vi "List ST-Link Infors.vi"(8 "error in (no error)":errorcluster) -> (0 "error out":errorcluster, 2 "Number":i32, 3 "ST-Links":cluster{"SN":string, "FW":string}[](array[cluster]))   [LabVIEW 2015, in "ST-Link.lvlib"]
doc: "识别已连接的ST-Link烧录器，返回连接数量，并获取其SN和FW版本信息。\n\n[ST-Links]: 簇数组，簇中包含两个元素。\n -->SN: 烧录器的SN；\n --> FW: 烧录器的固件版本；\n[Number]: 返回连接的烧录器数量。"
uses:
  ST-Link.lvlib
panel:
  out "standard output":string
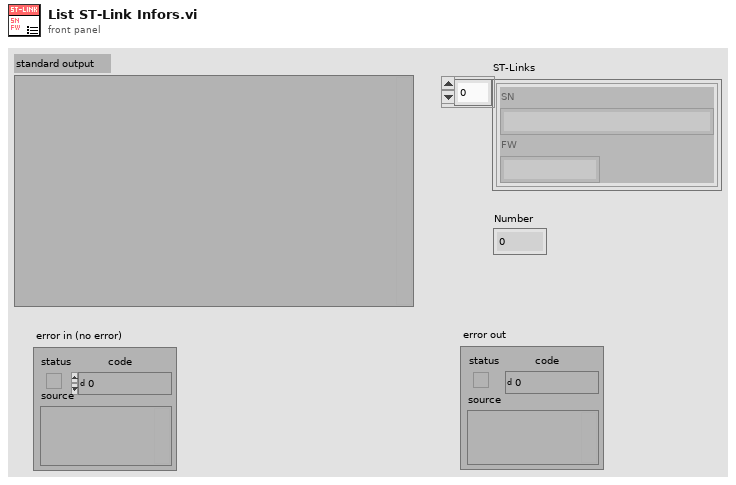
[diagram p1: front panel]
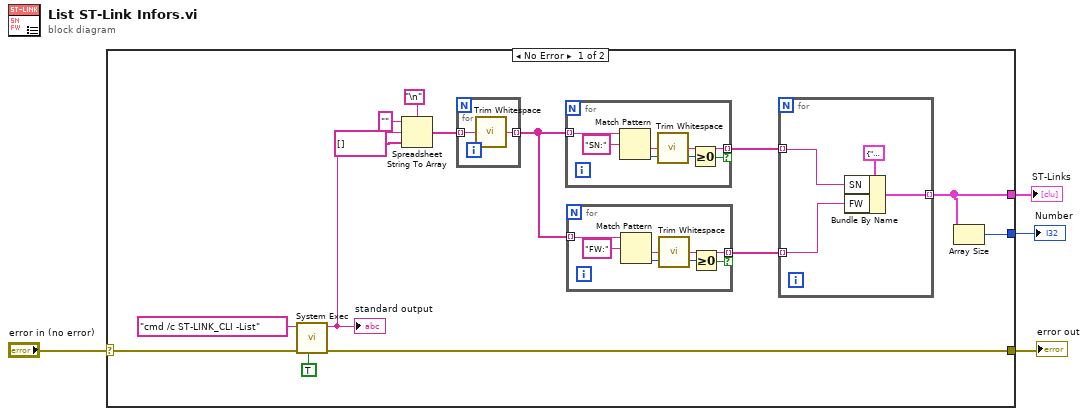
[diagram p0: block diagram]
diagram:
  n1 = case shown="No Error" "error in (no error)" {
    selector: "error in (no error)" -> [w16 w37]
    tunnel: [w15 w37] -> w3
    tunnel: [w6 _] -> w2
    tunnel: [w5 _] -> w1
    frame No Error {
      n2 = call <vilib>:"System Exec.vi"("run minimized? (F)"=TRUE, "error in (no error)"=w16, "command line"="cmd /c ST-LINK_CLI -List") -> ("error out"=w15:errorcluster, "standard output"=w9:string)  [unwired: 5 in, 2 out]
      "standard output" <- w9
      n3 = Spreadsheet String To Array(delimiter (Tab)="\n", format string="", spreadsheet string=w9, array type (2D Dbl)=string[] []) -> (array=w11:string[])
      n4 = for {
        tunnel: w11 -> [w36] mode=indexing
        tunnel: [w35] -> w10 mode=indexing
        n5 = call <vilib>:"Trim Whitespace.vi"("string"=w36) -> ("trimmed string"=w35:string)  [unwired: 1 in]
      }
      n6 = for {
        tunnel: w10 -> [w34] mode=indexing
        tunnel: [w29] -> w8 mode=indexing if=w30
        n7 = Match Pattern(string=w34, regular expression="SN:") -> (after substring=w32:string, offset past match=w31:i32)  [unwired: 1 in, 2 out]
        n8 = call <vilib>:"Trim Whitespace.vi"("string"=w32) -> ("trimmed string"=w29:string)  [unwired: 1 in]
        n9 = Greater Or Equal To 0?(x=w31) -> (x >= 0?=w30:bool)
      }
      n10 = for {
        tunnel: w10 -> [w28] mode=indexing
        tunnel: [w23] -> w7 mode=indexing if=w24
        n11 = Match Pattern(string=w28, regular expression="FW:") -> (after substring=w26:string, offset past match=w25:i32)  [unwired: 1 in, 2 out]
        n12 = call <vilib>:"Trim Whitespace.vi"("string"=w26) -> ("trimmed string"=w23:string)  [unwired: 1 in]
        n13 = Greater Or Equal To 0?(x=w25) -> (x >= 0?=w24:bool)
      }
      n14 = for {
        tunnel: w8 -> [w21] mode=indexing
        tunnel: w7 -> [w20] mode=indexing
        tunnel: [w19] -> w6 mode=indexing
        n15 = Bundle By Name(cluster=cluster{"SN":string, "FW":string} {"SN"="", "FW"=""} ("ST-Link"), "SN"=w21, "FW"=w20) -> (w19:cluster{"SN":string, "FW":string})
      }
      n16 = Array Size(array=w6) -> (size(s)=w5:i32)
    }
    frame Error {
    }
  }
  "error out" <- w3
  "ST-Links" <- w2
  "Number" <- w1
